vi "Validate Measurement Client Name.vi"(8 "error in":errorcluster, 10 "requested plugin name":string, 11 "project ref":refnum<vi>) -> (0 "error out":errorcluster, 3 "valid name?":bool)   [LabVIEW 2021, in "Create Measurement Plug-In Client.lvlib"]
uses:
  48953c88-0603-4c13-ba6a-df914321b09e.vi
  <vilib>/Comparison/Equal/Equal Functor/Equal Functor.lvclass
  Create Measurement Plug-In Client.lvlib
panel:
  out "control chars":string
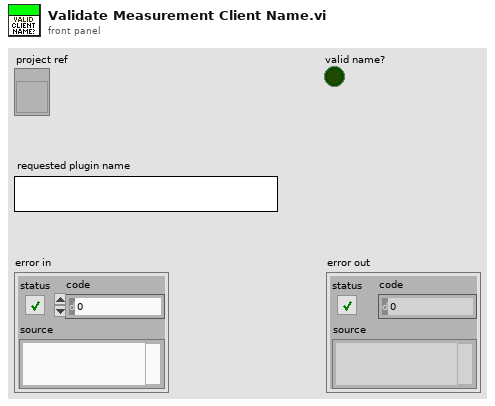
[diagram p1: front panel]
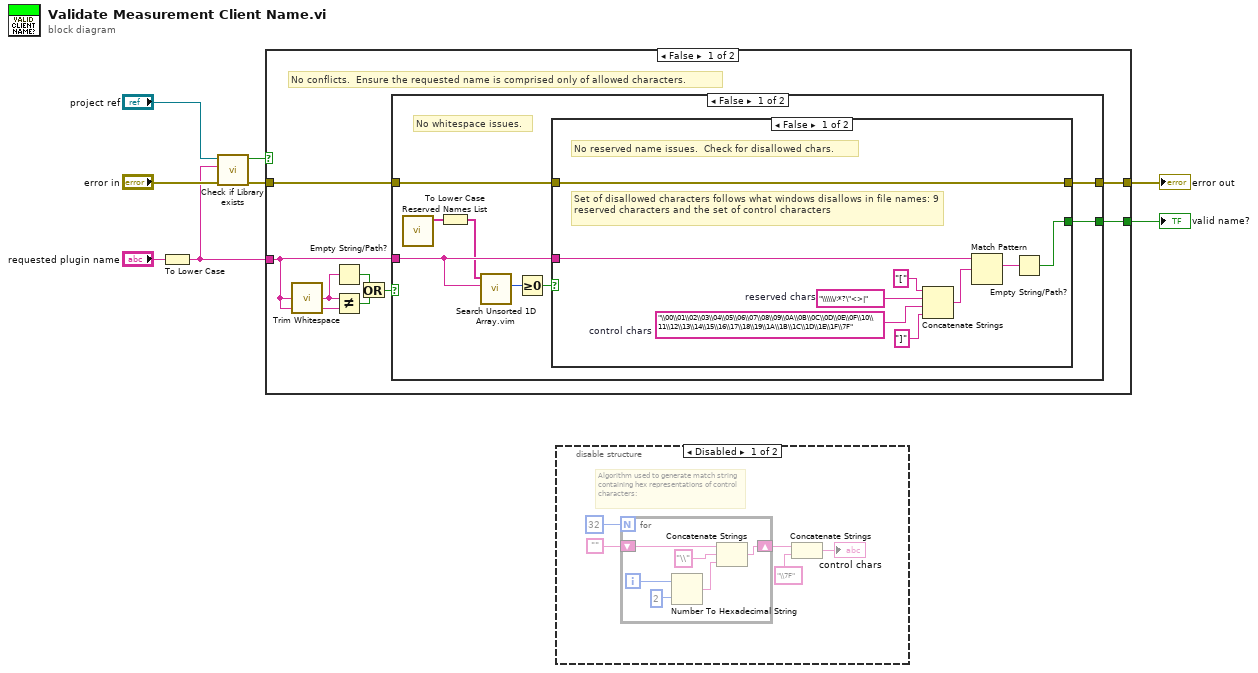
[diagram p0: block diagram]
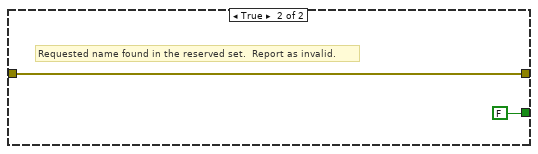
[diagram p3: hidden frame]
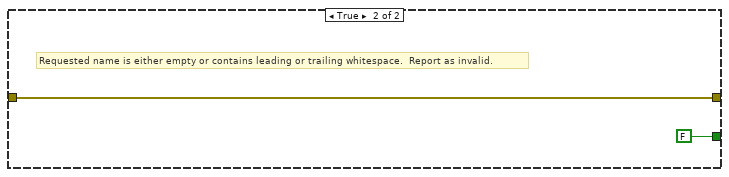
[diagram p4: hidden frame]
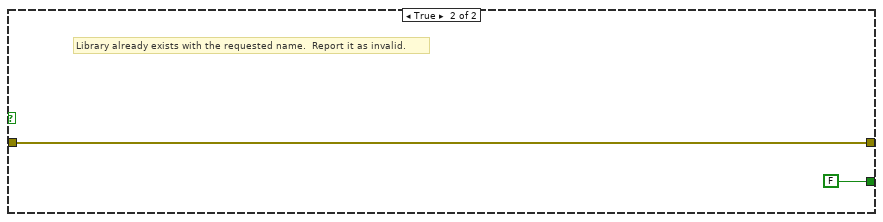
[diagram p5: hidden frame]
diagram:
  n1 = To Lower Case(string="requested plugin name") -> (all lower case string=w1:string)
  n2 = call "Check if Library exists.vi"("error in (no error)"="error in", "library name"=w1, "project ref"="project ref") -> ("error out"=w5:errorcluster, "found"=w6:bool)  [unwired: 7 in]
  n3 = case shown="False" w6 {
    tunnel: w5 -> [w16 w39]
    tunnel: [w15 w39] -> w4
    tunnel: [w14 FALSE ("Valid Name?")] -> w3
    tunnel: w1 -> [w9 _]
    frame False {
      # "No conflicts.  Ensure the requested name is comprised only of allowed characters."
      n4 = call <vilib>:"Trim Whitespace.vi"("string"=w9) -> ("trimmed string"=w13:string)  [unwired: 1 in]
      n5 = Empty String/Path?(string/path=w13) -> (empty?=w11:bool)
      n6 = Not Equal?(x=w13, y=w9) -> (x != y?=w12:bool)
      n7 = Or(x=w11, y=w12) -> (x .or. y?=w10:bool)
      n8 = case shown="False" w10 {
        tunnel: w9 -> [w19 _]
        tunnel: w16 -> [w24 w37]
        tunnel: [w23 w37] -> w15
        tunnel: [w20 FALSE ("Error if not Found (T)")] -> w14
        frame False {
          # "No whitespace issues."
          n9 = call "Reserved Names List.vi"() -> ("reserved names"=w18:string[])  [unwired: 11 in]
          n10 = To Lower Case(string=w18) -> (all lower case string=w17:string[])
          n11 = call "Search Unsorted 1D Array.vim"("element"=w19, "unsorted 1D array"=w17) -> ("index of element"=w22:i32)  [unwired: 9 in]
          n12 = Greater Or Equal To 0?(x=w22) -> (x >= 0?=w21:bool)
          n13 = case shown="False" w21 {
            tunnel: w19 -> [w32 _]
            tunnel: w24 -> [w33 w35]
            tunnel: [w33 w35] -> w23
            tunnel: [w30 FALSE ("Error if not Found (T)")] -> w20
            frame False {
              w25 = "\\00\\01\\02\\03\\04\\05\\06\\07\\08\\09\\0A\\0B\\0C\\0D\\0E\\0F\\10\\11\\12\\13\\14\\15\\16\\17\\18\\19\\1A\\1B\\1C\\1D\\1E\\1F\\7F"  # control chars
              w29 = "\\\\\\/:*?\"<>|"  # reserved chars
              # "Set of disallowed characters follows what windows disallows in file names: 9 reserved characters and the set of control characters"
              # "No reserved name issues.  Check for disallowed chars."
              n14 = Concatenate Strings("[" ("string"), w29, w25, "]" ("string")) -> (w26:string)
              n15 = Match Pattern(string=w32, regular expression=w26) -> (match substring=w31:string)  [unwired: 1 in, 3 out]
              n16 = Empty String/Path?(string/path=w31) -> (empty?=w30:bool)
            }
            frame True {
              # "Requested name found in the reserved set.  Report as invalid."
            }
          }
        }
        frame True {
          # "Requested name is either empty or contains leading or trailing whitespace.  Report as invalid."
        }
      }
    }
    frame True {
      # "Library already exists with the requested name.  Report it as invalid."
    }
  }
  "error out" <- w4
  "valid name?" <- w3
  n17 = disable-structure shown="Disabled" {
    frame Disabled {
      # "Algorithm used to generate match string containing hex representations of control characters:"
      n18 = for {
        N: 32 -> [_]
        shift-right: [w46] -> w42
        shift-left: "" -> [w45]
        i -> [w50]
        n19 = Number To Hexadecimal String(1:i16 2 ("width (-)"), 2:w50) -> (0:w48:string)
        n20 = Concatenate Strings(w45, "\\" ("string"), w48) -> (w46:string)
      }
      n21 = Concatenate Strings(w42, "\\7F") -> (→"control chars":string)
    }
    frame Enabled {
    }
  }
